vi "Resize Image.vi"   [LabVIEW 2020, in "G-Image.lvlib"]
doc: "<b>This VI is polymorphic.</b>\n\nResize the input image by the specified width and height, or by a scale multiplier.\n\n<b>Filter</b> sets the filter type used when resizing. When set to Default, the Catmull-Rom filter is used when upsampling images, and the Mitchell filter used when downsampling images.\n\n<b>Note:</b> 8-bit images will be converted to true color images when resized."
uses:
  G-Image.lvlib
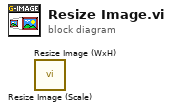
[diagram p0: block diagram]
diagram:
  n1 = call "Resize Image (Scale).vi"() -> ()  [unwired: 10 in, 2 out]
  n2 = call "Resize Image (WxH).vi"() -> ()  [unwired: 10 in, 2 out]
